vi "Periodic Tasks.vi"(8 "error in":errorcluster) -> ()   [LabVIEW 2016]
doc: "This VI runs in parallel to other tasks. It can contain as many user-defined periodic loops as you need. These can carry out PID or other sorts of timed response."
uses:
  <vilib>/Platform/TimedLoop/XDataNode/timing_clust.ctl
  <vilib>/Platform/TimedLoop/XDataNode/nitl_modes.ctl
  <vilib>/Platform/TimedLoop/XDataNode/wakeup.ctl
  <vilib>/platform/TimedLoop/XDataNode/XDataNode.xnode
  <vilib>/Platform/TimedLoop/XDataNode/XDNodeRunTimeDep.lvlib
panel:
  out "Numeric 5":dbl
  out "Numeric 4":dbl
  in  "Numeric 3":u8
  in  "Enum":T1(ring)
  in  "Numeric":u8
  in  "Numeric 2":u8
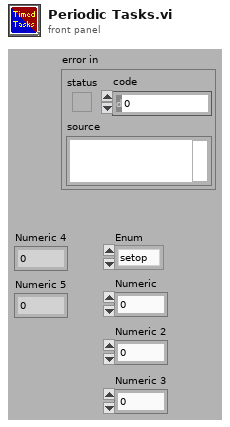
[diagram p1: front panel]
types:
  T1 = enum8{"setop", "setcolor", "default", "pilot", "ball", "gear", "both", "gearDeliver", "timeWarn", "targeting", "rave", "debug", ""}
  T2 = typedef "WPI_I2CDevRef.ctl" = cluster{"DevStatus":errorcluster, "Device Address":u8, "Handle":i32, "I2C Bus":T3}
  T3 = typedef "i2c_bus.ctl" = enum16{"I2C On-Board", "I2C MXP", "Invalid"}
  T4 = typedef "XDNodeRunTimeDep.lvlib/timing_clust.ctl" = cluster{"Expected End [f-1]":u64, "Actual End [f-1]":u64, "Finished Late? [f-1]":bool, "Expected End [i-1]":u64, "Actual End [i-1]":u64, "Finished Late? [i-1]":bool, "Expected Start [i]":u64, "Actual Start [i]":u64, "Expected Start [f]":u64, "Actual Start [f]":u64, "Source Name":string, "Structure Name":string, "Period":i64, "Deadline":i64, "Offset":i64, "Start":i64, "Priority":i32, "Timeout":i32, "Mode":T5, "Wakeup Reason":T6, "Error":errorcluster, "Source Type":string, "Secondary Source Type":string, "Global End Time":u64, "Global Start Time":u64, "Frame Duration":u64, "Iteration Duration":u64, "Assigned CPU":i32, "I/O Scan Engine Mode":u32}
  T5 = typedef "XDNodeRunTimeDep.lvlib/nitl_modes.ctl" = enum32{"No Change", "Process missed periods, maintain original phase", "Discard missed periods, maintain original phase", "Process missed periods, ignore original phase", "Discard missed periods, ignore original phase"}
  T6 = typedef "XDNodeRunTimeDep.lvlib/wakeup.ctl" = enum32{"Normal", "Aborted", "Asynchronous wakeup", "Timing source error", "Timed loop error", "Timeout"}
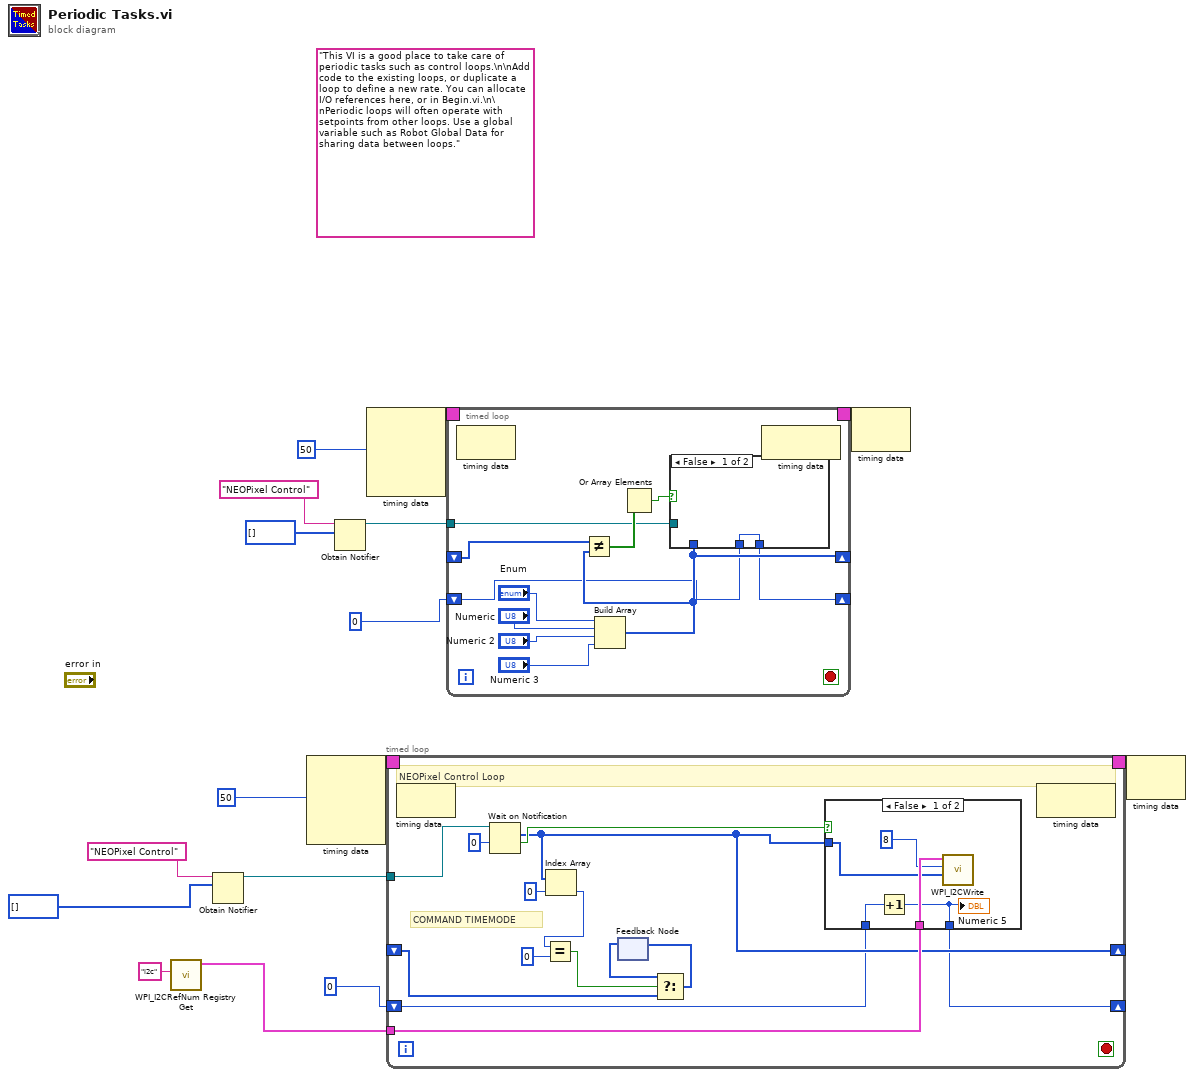
[diagram p0: block diagram]
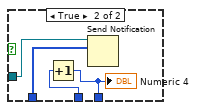
[diagram p3: hidden frame]
diagram:
  (unwired) "This VI is a good place to take care of periodic tasks such as control loops.\n\nAdd code to the existing loops, or duplicate a loop to define a new rate. You can allocate I/O references here, or in Begin.vi.\n\nPeriodic loops will often operate with setpoints from other loops. Use a global variable such as Robot Global Data for sharing data between loops."
  n1 = call <vilib>:"WPI_I2CRefNum Registry Get.vi"("refnum name"="i2c") -> ("I2CDevRef"=w4:T2)  [unwired: 9 in, 1 out]
  n2 = Obtain Notifier(name (unnamed)="NEOPixel Control", notification data type=u8[] []) -> (notifier out=w6:refnum<notifier>)  [unwired: 2 in, 2 out]
  n3 = node-c288(i64 50 ("Period")) -> (w10:T4)  [unwired: 3 in]
  n4 = Obtain Notifier(name (unnamed)="NEOPixel Control", notification data type=u8[] []) -> (notifier out=w13:refnum<notifier>)  [unwired: 2 in, 2 out]
  n5 = node-c288(i64 50 ("Period")) -> (w16:T4)  [unwired: 3 in]
  n6 = timed-loop {
    tunnel: w6 -> [w30]
    timing: w10 -> [_]
    timing-out: [_] -> w9
    tunnel: w4 -> [w27]
    shift-right: [w23] -> _
    shift-left: _ -> [w26]
    shift-right: [w17] -> _
    shift-left: 0 -> [w18]
    stop <- _ stop-if-true
    # "COMMAND TIMEMODE"
    # "NEOPixel Control Loop"
    n7 = node-c288() -> ()  [unwired: 1 in, 1 out]
    n8 = Wait on Notification(notifier=w30, timeout in ms (-1)=0) -> (notification=w23:u8[], timed out?=w28:bool)  [unwired: 2 in, 2 out]
    n9 = Index Array(array=w23, index=0) -> (element=w21:u8)
    n10 = Equal?(x=w21, y=u8 0) -> (x = y?=w19:bool)
    n11 = feedback #1() -> (w24:u8[])  [unwired: 1 in]
    n12 = Select(t=w24, s=w19, f=w26) -> (s? t:f=w25:u8[])
    n13 = feedback-in #1(w25) -> ()
    n14 = case shown="False" w28 {
      tunnel: w23 -> [w33 _]
      tunnel: w27 -> [w35 _]
      tunnel: w18 -> [w32 w36]
      tunnel: [w31 w36] -> w17
      frame False {
        n15 = Increment(x=w32) -> (x+1=w31:i32)
        "Numeric 5" <- w31
        n16 = call <vilib>:"WPI_I2CWrite.vi"("I2CDataToSend"=w33, "I2CRegister"=u8 8, "I2CDevRef"=w35) -> ()  [unwired: 7 in, 2 out]
      }
      frame True {
      }
    }
    n17 = node-c288() -> ()  [unwired: 1 in, 1 out]
  }
  n18 = timed-loop {
    timing: w16 -> [_]
    timing-out: [_] -> w15
    shift-right: [w45] -> _
    shift-left: _ -> [w44]
    tunnel: w13 -> [w41]
    shift-right: [w39] -> _
    shift-left: 0 -> [w40]
    stop <- _ stop-if-true
    n19 = node-c288() -> ()  [unwired: 1 in, 1 out]
    n20 = Build Array("Enum", "Numeric", "Numeric 2", "Numeric 3") -> (w45:u8[])
    n21 = Not Equal?(x=w44, y=w45) -> (x != y?=w43:bool[])
    n22 = Or Array Elements(Boolean array=w43) -> (logical OR=w42:bool)
    n23 = case shown="False" w42 {
      tunnel: w45 -> [_ w54]
      tunnel: w41 -> [_ w53]
      tunnel: w40 -> [w50 w52]
      tunnel: [w50 w51] -> w39
      frame False {
      }
      frame True {
        n24 = Increment(x=w52) -> (x+1=w51:i32)
        "Numeric 4" <- w51
        n25 = Send Notification(notification=w54, notifier=w53) -> ()  [unwired: 1 in, 2 out]
      }
    }
    n26 = node-c288() -> ()  [unwired: 1 in, 1 out]
  }
  n27 = node-c288(w15) -> ()  [unwired: 1 out]
  n28 = node-c288(w9) -> ()  [unwired: 1 out]
